vi "Phasor Correct Complex Phasor (Calibration Map) v3.vi"(7 "Calibration Phasor":T1, 8 "Error In":errorcluster, 10 "Phasor Calibration Map":T2={"Phasor Frequency"=80000000.0, "Calibration Lifetime"=1e-09, "ROI Centers"=[], "ROI Descriptors"=[], "Map Resolution X"=0, "Map Resolution Y"=0, "z Array"=[]} {"ROI Descriptors"."Contours"."Type" items=["No Selection", "Point", "Line", "Rectangle", "Oval", "Polygon", "Freehand Region", "Annulus", "Unused2", "Unused3", "Broken Line", "Freehand Line", "Rotated Rectangle"]}, 11 "Complex Phasor Array (VxH)":csg[][](array[numeric])) -> (0 "Error Out":errorcluster, 3 "Corrected Complex Phasor Array (VxH)":csg[][](array[numeric]), 6 "CPU (s)":dbl)   [LabVIEW 2021, in "Phasor.lvlib"]
uses:
  Phasor.lvlib
  Phasor Calibration Map v2.ctl
  Calibration Phasor (m, phi).ctl
  fc03083e-373a-4876-b88b-03b42af37d1f.vi
  16d35b92-a371-4f93-9997-5685d56f4b99.vi
  8b925e9c-e4c5-4623-82c6-9f66945b4c7b.vi
  Time/Time.lvlib
  Utilities/Utilities.lvlib
panel:
  out "Map presorting (s)":dbl
  out "Calibration Map Search (s)":dbl
  # "see the License on the block diagram (Ctrl+E or Window:Show Block Diagram)"
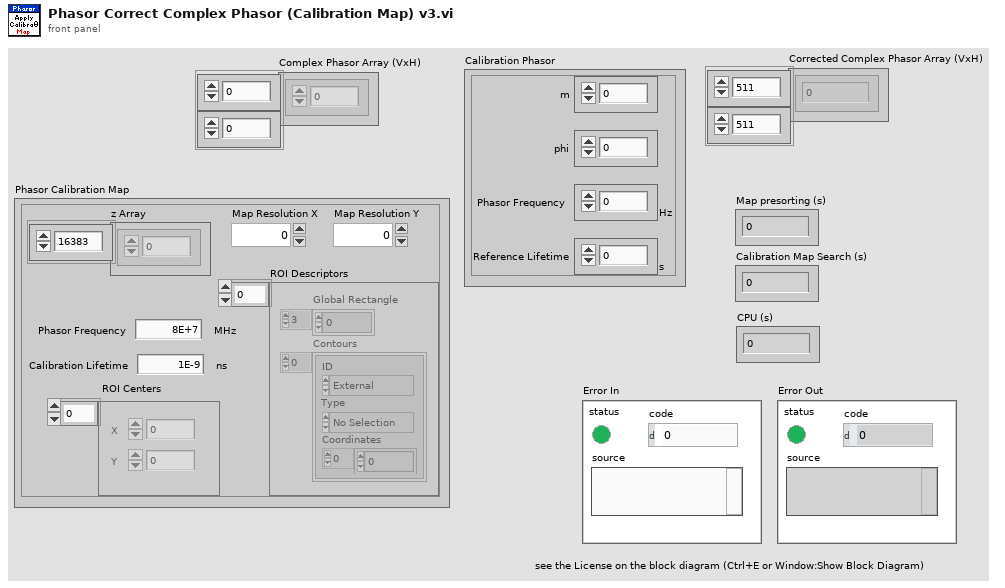
[diagram p1: front panel]
types:
  T1 = typedef "Phasor.lvlib/Calibration Phasor (m, phi).ctl" = cluster{"m":dbl, "phi":dbl, "Phasor Frequency":dbl[unit], "Reference Lifetime":dbl[unit]}
  T2 = typedef "Phasor.lvlib/Phasor Calibration Map v2.ctl" = cluster{"Phasor Frequency":dbl[unit], "Calibration Lifetime":dbl[unit], "ROI Centers":cluster{"X":i32, "Y":i32}[], "ROI Descriptors":T3[], "Map Resolution X":i32, "Map Resolution Y":i32, "z Array":cdb[]}
  T3 = typedef "ROI Descriptor" = cluster{"Global Rectangle":i32[], "Contours":cluster{"ID":enum32{"External", "Internal"}, "Type":u32, "Coordinates":i32[]}[]}
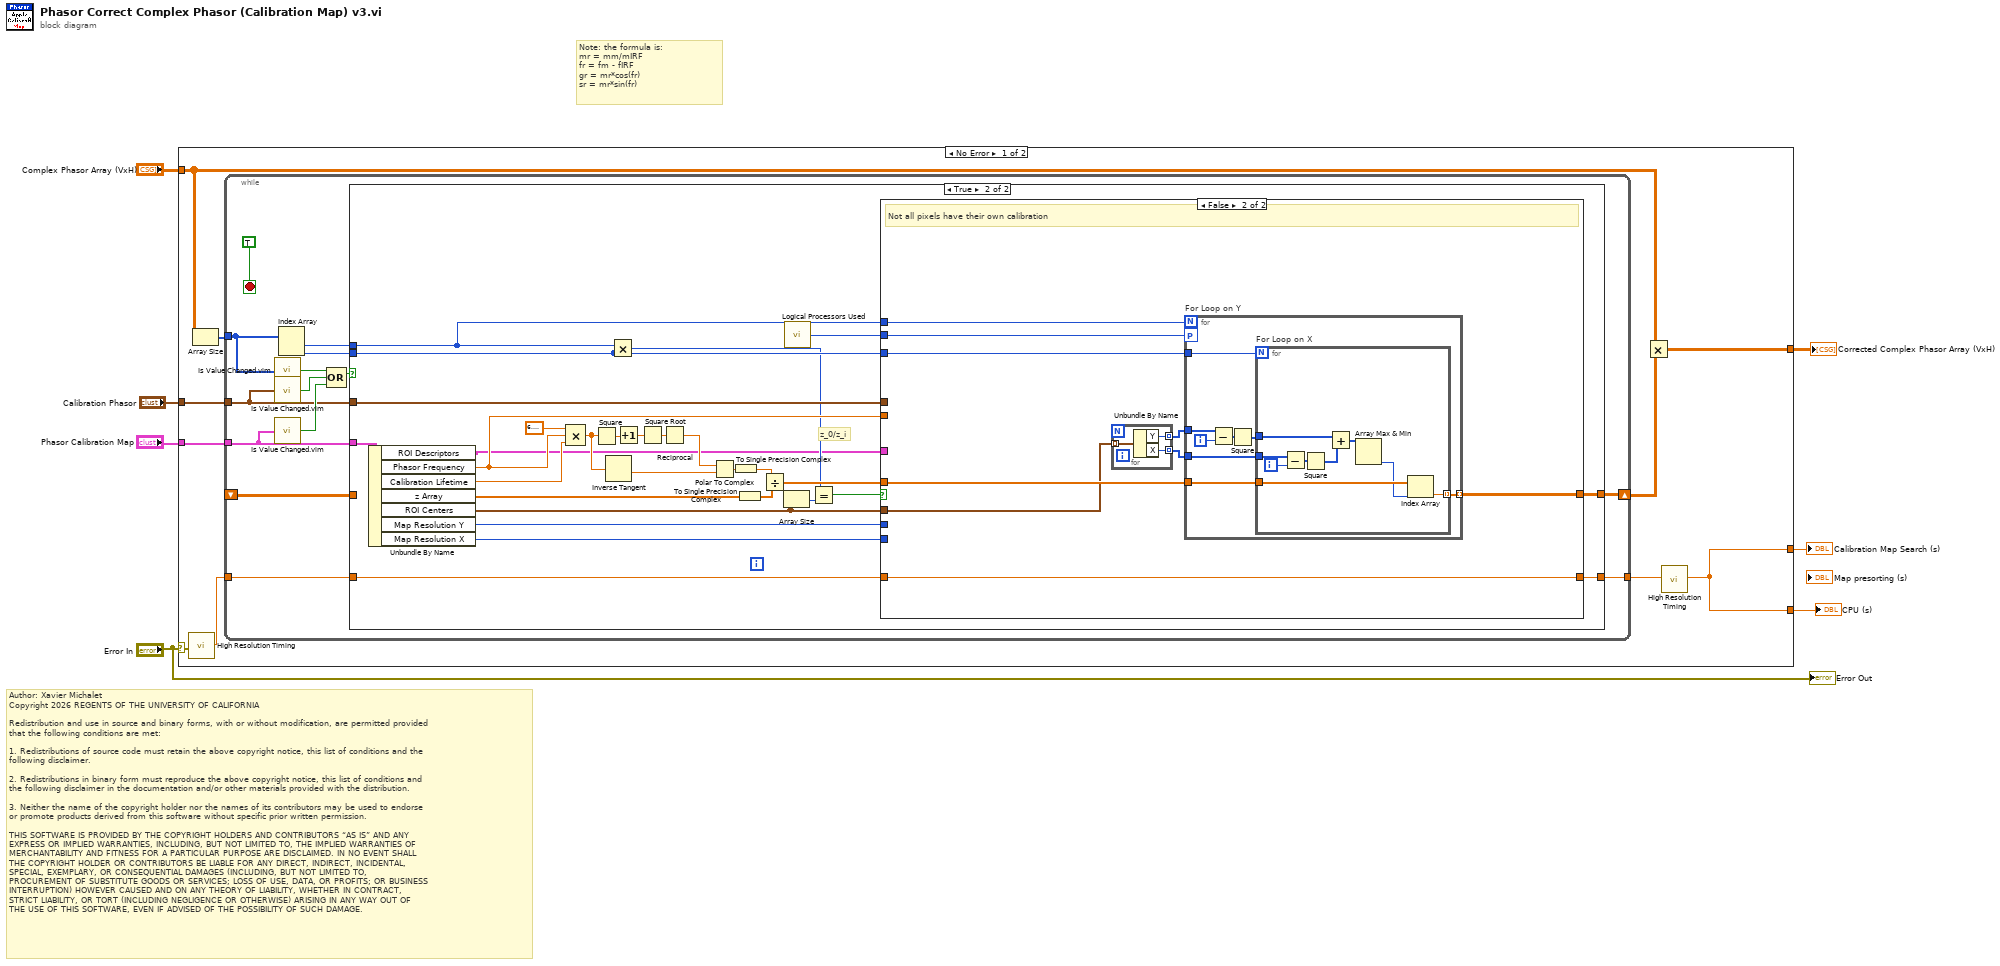
[diagram p0: block diagram]
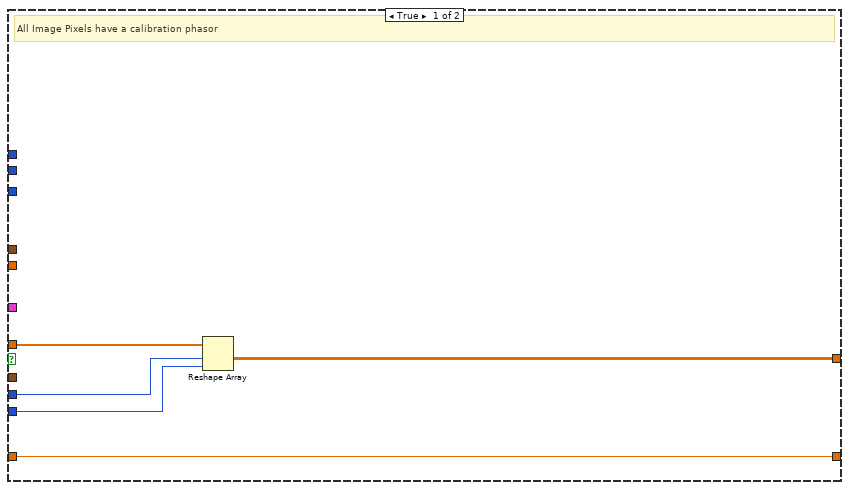
[diagram p3: hidden frame]
diagram:
  # "Author: Xavier Michalet\nCopyright 2026 REGENTS OF THE UNIVERSITY OF CALIFORNIA\n\nRedistribution and use in source and binary forms, with or without modification, are permitted provided\nthat the following conditions are met:\n\n1. Redistributions of source code must retain the above copyright notice, this list of conditions and the\nfollowing disclaimer.\n\n2. Redistributions in binary form must reproduce the above copyright notice, this list of conditions and\nthe following disclaimer in the documentation and/or other materials provided with the distribution.\n\n3. Neither the name of the copyright holder nor the names of its contributors may be used to endorse \nor promote products derived from this software without specific prior written permission.\n\nTHIS SOFTWARE IS PROVIDED BY THE COPYRIGHT HOLDERS AND CONTRIBUTORS “AS IS” AND ANY \nEXPRESS OR IMPLIED WARRANTIES, INCLUDING, BUT NOT LIMITED TO, THE IMPLIED WARRANTIES OF\nMERCHANTABILITY AND FITNESS FOR A PARTICULAR PURPOSE ARE DISCLAIMED. IN NO EVENT SHALL\nTHE COPYRIGHT HOLDER OR CONTRIBUTORS BE LIABLE FOR ANY DIRECT, INDIRECT, INCIDENTAL, \nSPECIAL, EXEMPLARY, OR CONSEQUENTIAL DAMAGES (INCLUDING, BUT NOT LIMITED TO, \nPROCUREMENT OF SUBSTITUTE GOODS OR SERVICES; LOSS OF USE, DATA, OR PROFITS; OR BUSINESS\nINTERRUPTION) HOWEVER CAUSED AND ON ANY THEORY OF LIABILITY, WHETHER IN CONTRACT, \nSTRICT LIABILITY, OR TORT (INCLUDING NEGLIGENCE OR OTHERWISE) ARISING IN ANY WAY OUT OF\nTHE USE OF THIS SOFTWARE, EVEN IF ADVISED OF THE POSSIBILITY OF SUCH DAMAGE."
  # "Note: the formula is:\nmr = mm/mIRF\nfr = fm - fIRF\ngr = mr*cos(fr)\nsr = mr*sin(fr)"
  n1 = case shown="No Error" "Error In" {
    selector: "Error In" -> [w12 _]
    tunnel: [w17 w97] -> w7
    tunnel: "Phasor Calibration Map" -> [w16 _]
    tunnel: [w9 _] -> w5
    tunnel: "Complex Phasor Array (VxH)" -> [w15 w97]
    tunnel: [w9 _] -> w3
    tunnel: "Calibration Phasor" -> [w11 _]
    frame No Error {
      n2 = call "High Resolution Timing.vi"("Error In"=w12) -> ("elapsed (relative) seconds"=w8:dbl)  [unwired: 16 in, 2 out]
      n3 = Array Size(array=w15) -> (size(s)=w10:i32[])
      n4 = while {
        tunnel: w16 -> [w23]
        tunnel: w8 -> [w26]
        tunnel: w10 -> [w19]
        shift-right: [w30] -> w14
        shift-left: _ -> [w24]
        tunnel: [w25] -> w13
        tunnel: w11 -> [w21]
        stop <- TRUE stop-if-true
        n5 = call "Is Value Changed.vim"("value"=w19) -> ("changed or first call?"=w18:bool)
        n6 = call "Is Value Changed.vim"("value"=w21) -> ("changed or first call?"=w20:bool)
        n7 = call "Is Value Changed.vim"("value"=w23) -> ("changed or first call?"=w22:bool)
        n8 = Index Array(array=w19) -> (element #1=w28:i32, element #2=w27:i32)  [unwired: 2 in]
        n9 = Compound Arithmetic op=OR(w18, w20, w22) -> (w29:bool)
        n10 = case shown="True" w29 {
          tunnel: [w33 w58] -> w30
          tunnel: w24 -> [w33 _]
          tunnel: w28 -> [_ w39]
          tunnel: w27 -> [_ w38]
          tunnel: w23 -> [_ w57]
          tunnel: w26 -> [w32 w56]
          tunnel: [w32 w55] -> w25
          tunnel: w21 -> [_ w44]
          frame False {
          }
          frame True {
            # "z_0/z_i"
            n11 = Unbundle By Name(w57) -> ("ROI Descriptors"=w35:T3[], "Phasor Frequency"=w43:dbl[unit], "Calibration Lifetime"=w62:dbl[unit], "z Array"=w61:cdb[], "ROI Centers"=w40:cluster{"X":i32, "Y":i32}[], "Map Resolution Y"=w42:i32, "Map Resolution X"=w41:i32)
            n12 = Compound Arithmetic op=MULTIPLY(6.283185307179586, w43, w62) -> (w53:dbl)
            n13 = Square(x=w53) -> (x^2=w52:dbl)
            n14 = Inverse Tangent(1:w53) -> (0:w50:dbl)
            n15 = Multiply(x=w39, y=w38) -> (x*y=w36:i32)
            n16 = Increment(x=w52) -> (x+1=w51:dbl)
            n17 = Square Root(x=w51) -> (sqrt(x)=w49:dbl)
            n18 = Reciprocal(x=w49) -> (1/x=w48:dbl)
            n19 = Polar To Complex(1:w50, 2:w48) -> (0:w47:cdb)
            n20 = To Single Precision Complex(1:w47) -> (0:w46:csg)
            n21 = To Single Precision Complex(1:w61) -> (0:w45:csg[])
            n22 = Divide(x=w46, y=w45) -> (x/y=w59:csg[])
            n23 = Array Size(array=w40) -> (size(s)=w37:i32)
            n24 = call "Logical Processors Used.vi"() -> ("# Logical Processor Used"=w60:i32)  [unwired: 6 in]
            n25 = Equal?(x=w36, y=w37) -> (x = y?=w34:bool)
            n26 = case shown="False" w34 {
              tunnel: w60 -> [_ w76]
              tunnel: w59 -> [w67 w75]
              tunnel: [w66 w74] -> w58
              tunnel: w39 -> [_ w73]
              tunnel: w38 -> [_ w72]
              tunnel: w40 -> [_ w71]
              tunnel: w56 -> [w65 w70]
              tunnel: [w65 w70] -> w55
              tunnel: w44 -> [_ _]
              tunnel: w43 -> [_ _]
              tunnel: w42 -> [w64 _]
              tunnel: w41 -> [w63 _]
              tunnel: w35 -> [_ _]
              frame True {
                # "All Image Pixels have a calibration phasor"
                n27 = Reshape Array(w67, w64, w63) -> (w66:csg[][])
              }
              frame False {
                # "Not all pixels have their own calibration"
                n28 = for {
                  tunnel: w71 -> [w79] mode=indexing
                  tunnel: [w78] -> w69 mode=indexing
                  tunnel: [w77] -> w68 mode=indexing
                  n29 = Unbundle By Name(w79) -> ("Y"=w78:i32, "X"=w77:i32)
                }
                n30 = for "For Loop on Y" {
                  N: w73 -> [_]
                  tunnel: w72 -> [w87]
                  tunnel: w69 -> [w84]
                  tunnel: w68 -> [w83]
                  workers-P: w76 -> [_]
                  tunnel: w75 -> [w81]
                  tunnel: [w80] -> w74 mode=indexing
                  i -> [w85]
                  n31 = Subtract(x=w84, y=w85) -> (x-y=w86:i32[])
                  n32 = Square(x=w86) -> (x^2=w82:i32[])
                  n33 = for "For Loop on X" {
                    N: w87 -> [_]
                    tunnel: w83 -> [w92]
                    tunnel: w82 -> [w91]
                    tunnel: w81 -> [w90]
                    tunnel: [w89] -> w80 mode=indexing
                    i -> [w93]
                    n34 = Subtract(x=w92, y=w93) -> (x-y=w96:i32[])
                    n35 = Square(x=w96) -> (x^2=w95:i32[])
                    n36 = Add(x=w91, y=w95) -> (x+y=w94:i32[])
                    n37 = Array Max & Min(array=w94) -> (min index (indices)=w88:i32)  [unwired: 3 out]
                    n38 = Index Array(array=w90, index=w88) -> (element=w89:csg)
                  }
                }
              }
            }
          }
        }
      }
      n39 = Multiply(x=w15, y=w14) -> (x*y=w17:csg[][])
      n40 = call "High Resolution Timing.vi"("relative seconds (NaN)"=w13) -> ("elapsed (relative) seconds"=w9:dbl)  [unwired: 16 in, 2 out]
    }
    frame Error {
    }
  }
  "Corrected Complex Phasor Array (VxH)" <- w7
  "Calibration Map Search (s)" <- w5
  "CPU (s)" <- w3
  "Error Out" <- "Error In"
